vi "Status Size.vi"(8 "error in (no error)":errorcluster) -> (0 "error out":errorcluster, 3 "size":u64)   [LabVIEW 2017, in "DSF Core.lvlib" / "Transfer Group Status.lvclass"]
uses:
  Transfer Group Status.lvclass
  Typedefs/DSF Transfer Group Status.ctl
  DSF Core.lvlib
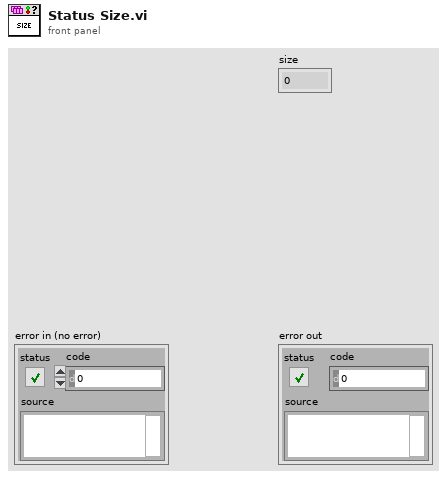
[diagram p1: front panel]
types:
  T1 = typedef "DSF Core.lvlib/DSF Transfer Group Status.ctl" = cluster{"late count":u64, "iteration":u64}
  T2 = enum16{"big-endian, network order", "native, host order", "little-endian"}
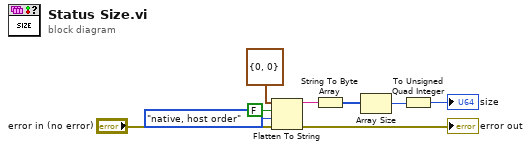
[diagram p0: block diagram]
diagram:
  n1 = Flatten To String(anything=T1 {"late count"=0, "iteration"=0} ("Transfer Group status"), prepend array or string size? (T)=FALSE, byte order (0:big-endian, network order)=T2."native, host order", error in (no error)="error in (no error)") -> (data string=w7:string, error out=→"error out":errorcluster)  [unwired: 1 out]
  n2 = String To Byte Array(string=w7) -> (unsigned byte array=w6:u8[])
  n3 = Array Size(array=w6) -> (size(s)=w5:i32)
  n4 = To Unsigned Quad Integer(1:w5) -> (0:→"size":u64)
